vi "RandomPOI.vi"(9 "Field of View":u16(ring) items=["130", "175", "260"], 10 "Objective":u16(ring)=1 items=["25X", "40X"], 11 "ZPlanes":dbl[](array[numeric]) format="%_6g") -> (3 "RandomPOI":i32[][](array[numeric]))   [LabVIEW 2017]
panel:
  in  "#POIs":i16=30
  in  "Nvox":i32=200
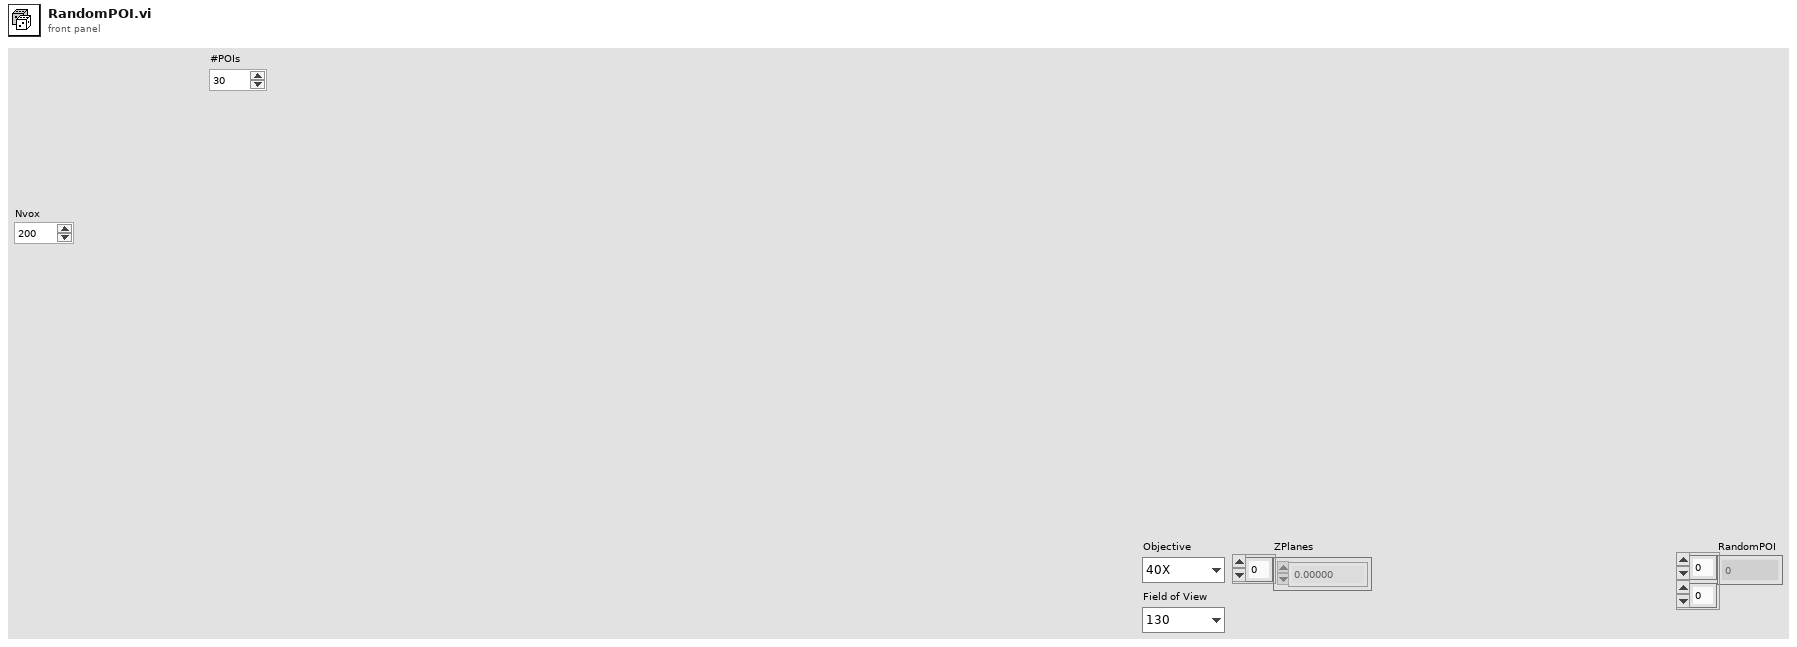
[diagram p1: front panel]
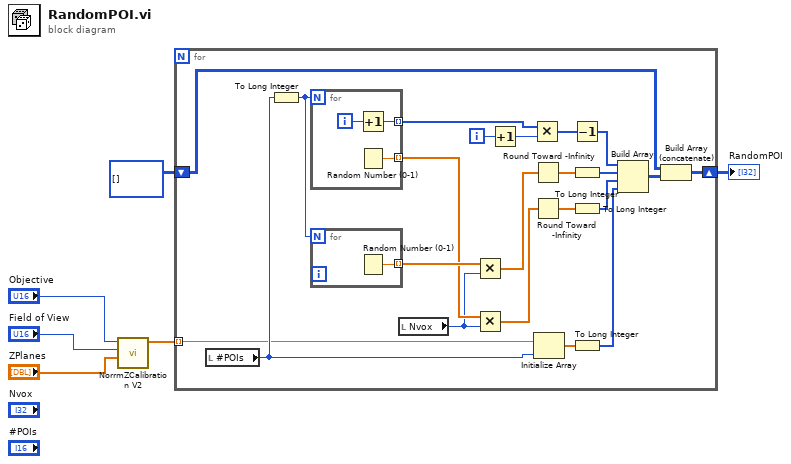
[diagram p0: block diagram]
diagram:
  n1 = call "NorrmZCalibration V2.vi"("xi"="ZPlanes", "Field of View"="Field of View", "Objective"="Objective") -> ("yi"=w5:dbl[])  [unwired: 6 in, 2 out]
  n2 = for {
    shift-right: [w16] -> w1
    shift-left: i32[][] [] -> [w15]
    tunnel: w5 -> [w10] mode=indexing
    i -> [w17]
    n3 = local read "#POIs"() -> (w26:i16)
    n4 = To Long Integer(number=w26) -> (32bit integer=w28:i32)
    n5 = for {
      N: w28 -> [_]
      tunnel: [w31] -> w23 mode=indexing
      tunnel: [w29] -> w18 mode=indexing
      i -> [w30]
      n6 = Increment(x=w30) -> (x+1=w29:i32)
      n7 = Random Number (0-1)() -> (number: 0 to 1=w31:dbl)
    }
    n8 = for {
      N: w28 -> [_]
      tunnel: [w32] -> w25 mode=indexing
      n9 = Random Number (0-1)() -> (number: 0 to 1=w32:dbl)
    }
    n10 = local read "Nvox"() -> (w22:i32)
    n11 = Multiply(x=w25, y=w22) -> (x*y=w27:dbl[])
    n12 = Multiply(x=w23, y=w22) -> (x*y=w24:dbl[])
    n13 = Increment(x=w17) -> (x+1=w12:i32)
    n14 = Multiply(x=w18, y=w12) -> (x*y=w13:i32[])
    n15 = Round Toward -Infinity(1:w27) -> (0:w19:dbl[])
    n16 = Round Toward -Infinity(1:w24) -> (0:w20:dbl[])
    n17 = Initialize Array(w10, w26) -> (w21:dbl[])
    n18 = Decrement(x=w13) -> (x-1=w11:i32[])
    n19 = To Long Integer(number=w19) -> (32bit integer=w9:i32[])
    n20 = To Long Integer(number=w20) -> (32bit integer=w8:i32[])
    n21 = To Long Integer(number=w21) -> (32bit integer=w7:i32[])
    n22 = Build Array(w11, w9, w8, w7) -> (w14:i32[][])
    n23 = Build Array (concatenate)(w15, w14) -> (w16:i32[][])
  }
  "RandomPOI" <- w1
